vi "XNET Convert (Signal to Frame Raw).vi"(0 "session in":refnum<k21>, 5 "signal data":dbl[](array[numeric]) format="%.2f", 11 "error in (no error)":errorcluster) -> (4 "session out":refnum<k21>, 6 "frame data":u8[](array[numeric]) format="%02x", 15 "error out":errorcluster)   [LabVIEW 2018]
doc: "Converts signal data to NI-XNET raw frame data."
uses:
  nixlvapi.dll
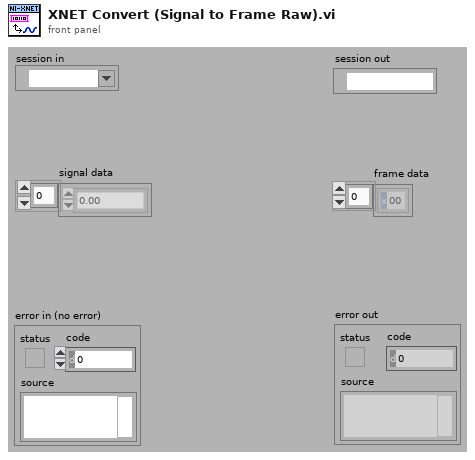
[diagram p1: front panel]
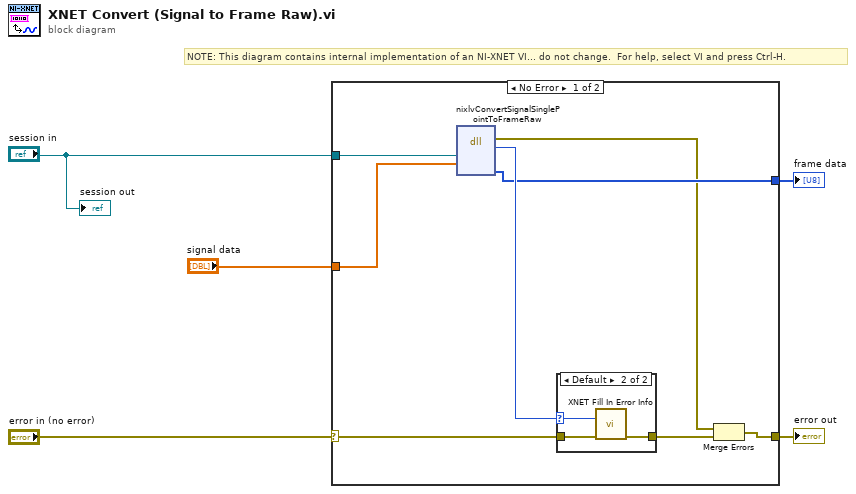
[diagram p0: block diagram]
diagram:
  # "NOTE: This diagram contains internal implementation of an NI-XNET VI... do not change.  For help, select VI and press Ctrl-H."
  n1 = case shown="No Error" "error in (no error)" {
    selector: "error in (no error)" -> [w12 w18]
    tunnel: "session in" -> [w13 _]
    tunnel: [w7 w18] -> w5
    tunnel: [w8 _] -> w2
    tunnel: "signal data" -> [w9 _]
    frame No Error {
      n2 = dll-call lib="nixlvapi.*" fn="nixlvConvertSignalSinglePointToFrameRaw"("sessionRef"=w13, "signalData"=w9) -> (error out=w6:errorcluster, "return type"=w10:i32, "frameData"=w8:u8[])  [unwired: 5 in, 2 out]
      n3 = case shown="Default" w10 {
        selector: w10 -> [_ w15]
        tunnel: w12 -> [w14 w16]
        tunnel: [w14 w17] -> w11
        frame 0 {
        }
        frame Default {
          n4 = call "XNET Fill In Error Info.vi"("status code"=w15, "error in"=w16) -> ("error out"=w17:errorcluster)  [unwired: 13 out]
        }
      }
      n5 = Merge Errors(w6, w11) -> (w7:errorcluster)
    }
    frame Error {
    }
  }
  "error out" <- w5
  "frame data" <- w2
  "session out" <- "session in"
